vi "Save Measurement.vi"(1 "Measurement Config":T1, 2 "Experiment Config":T2, 4 "DMM Value":dbl, 5 "DMM 2 Value":dbl, 6 "Diode PS Voltage":dbl, 7 "Diode PS Current":dbl, 8 "error in":errorcluster, 9 "Trace Number":u64, 10 "Measurement Timestamp":timestamp, 11 "Trace":waveform(dbl)) -> (0 "error out":errorcluster)   [LabVIEW 2020]
uses:
  Typedefs/Experiment Config Control.ctl
  Typedefs/Measurement Config.ctl
  <vilib>/Utility/file.llb/Write Delimited Spreadsheet (string).vi
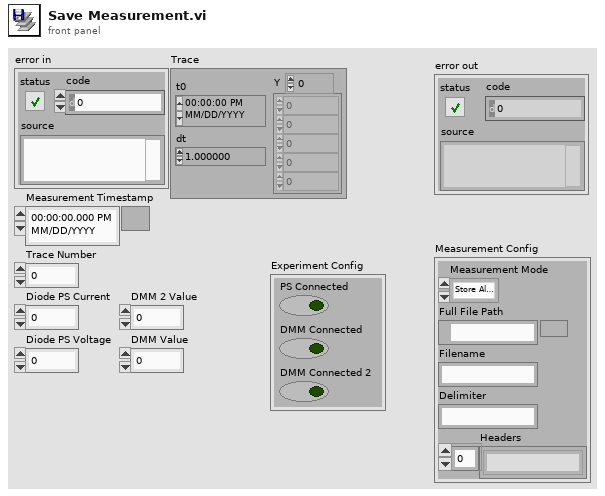
[diagram p1: front panel]
types:
  T1 = typedef "Measurement Config.ctl" = cluster{"Measurement Mode":enum16{"Store All Traces in Single File", "Store Average/Std. Dev. for each Point", "Store All Traces in Separate Files"}, "Full File Path":path, "Filename":string, "Delimiter":string, "Headers":string[]}
  T2 = typedef "Experiment Config Control.ctl" = cluster{"PS Connected":bool, "DMM Connected":bool, "DMM Connected 2":bool}
  T3 = enum16{"Store All Traces in Single File", "Store Average/Std. Dev. for each Point", "Store All Traces in Separate Files"}
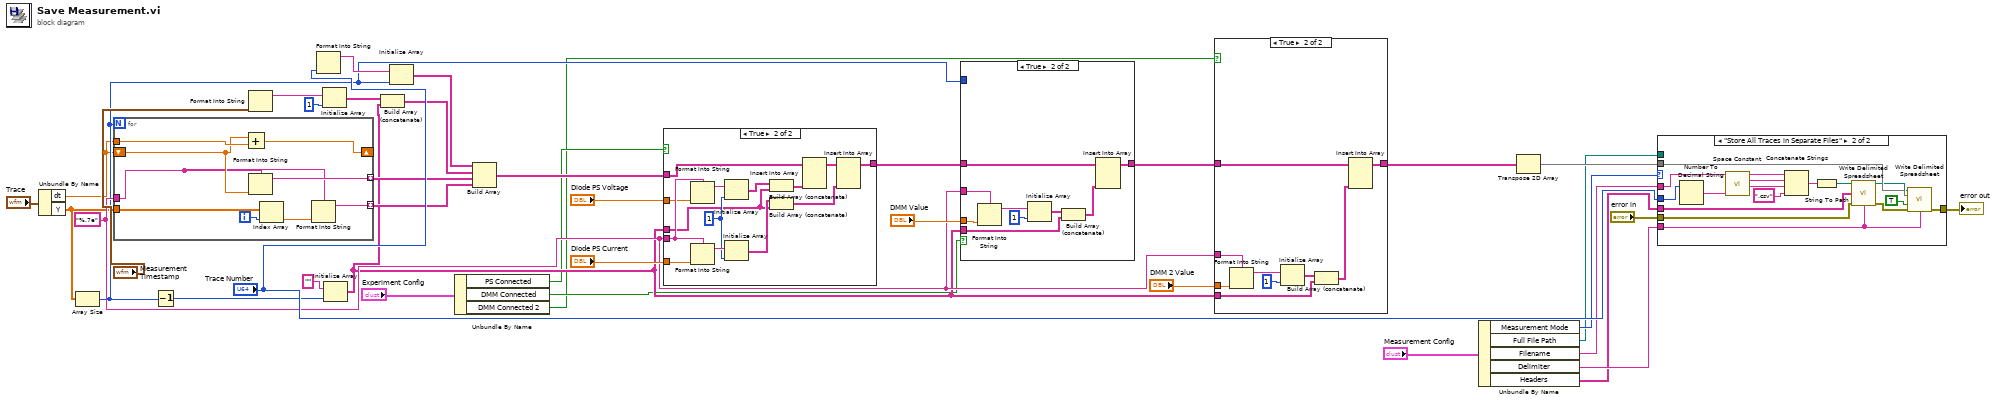
[diagram p0: block diagram]
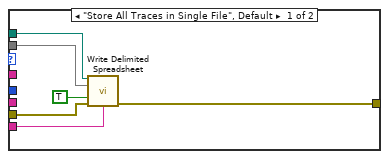
[diagram p3: hidden frame]
diagram:
  w17 = "%.7e"
  n1 = Unbundle By Name("Trace") -> ("dt"=w12:dbl, "Y"=w11:dbl[])
  n2 = Array Size(array=w11) -> (size(s)=w13:i32)
  n3 = for {
    N: w13 -> [_]
    shift-right: [w47] -> _
    shift-left: w12 -> [w46]
    tunnel: w12 -> [w48]
    tunnel: w11 -> [w42]
    tunnel: [w44] -> w26 mode=indexing
    tunnel: [w43] -> w27 mode=indexing
    tunnel: w17 -> [w40]
    i -> [w45]
    n4 = Add(x=w46, y=w48) -> (x+y=w47:dbl)
    n5 = Format Into String(format string=w40, w46) -> (resulting string=w43:string)  [unwired: 2 in, 1 out]
    n6 = Index Array(array=w42, index=w45) -> (element=w41:dbl)
    n7 = Format Into String(format string=w40, w41) -> (resulting string=w44:string)  [unwired: 2 in, 1 out]
  }
  n8 = Decrement(x=w13) -> (x-1=w21:i32)
  n9 = Format Into String("Measurement Timestamp") -> (resulting string=w29:string)  [unwired: 3 in, 1 out]
  n10 = Format Into String("Trace Number") -> (resulting string=w30:string)  [unwired: 3 in, 1 out]
  n11 = Initialize Array(w29, 1) -> (w19:string[])
  n12 = Initialize Array("", w21) -> (w16:string[])
  n13 = Build Array (concatenate)(w19, w16) -> (w18:string[])
  n14 = Initialize Array(w30, w13) -> (w28:string[])
  n15 = Unbundle By Name("Experiment Config") -> ("PS Connected"=w9:bool, "DMM Connected"=w8:bool, "DMM Connected 2"=w7:bool)
  n16 = Build Array(w28, w18, w27, w26) -> (w24:string[][])
  n17 = case shown="True" w9 {
    tunnel: w17 -> [_ w63]
    tunnel: "Diode PS Voltage" -> [_ w62]
    tunnel: "Diode PS Current" -> [_ w61]
    tunnel: w24 -> [w49 w58]
    tunnel: [w49 w56] -> w23
    tunnel: w16 -> [_ w50]
    frame False {
    }
    frame True {
      w55 = 1
      n18 = Format Into String(format string=w63, w62) -> (resulting string=w59:string)  [unwired: 2 in, 1 out]
      n19 = Format Into String(format string=w63, w61) -> (resulting string=w60:string)  [unwired: 2 in, 1 out]
      n20 = Initialize Array(w59, w55) -> (w54:string[])
      n21 = Initialize Array(w60, w55) -> (w52:string[])
      n22 = Build Array (concatenate)(w54, w50) -> (w53:string[])
      n23 = Build Array (concatenate)(w52, w50) -> (w51:string[])
      n24 = Insert Into Array(array=w58, new element=w53) -> (w57:string[][])  [unwired: 2 in]
      n25 = Insert Into Array(array=w57, new element=w51) -> (w56:string[][])  [unwired: 2 in]
    }
  }
  n26 = case shown="True" w8 {
    tunnel: w17 -> [_ w73]
    tunnel: "DMM Value" -> [_ w72]
    tunnel: w13 -> [_ _]
    tunnel: w23 -> [w64 w70]
    tunnel: [w64 w69] -> w15
    tunnel: w16 -> [_ w66]
    frame False {
    }
    frame True {
      n27 = Format Into String(format string=w73, w72) -> (resulting string=w71:string)  [unwired: 2 in, 1 out]
      n28 = Initialize Array(w71, 1 ("dimension size")) -> (w67:string[])
      n29 = Build Array (concatenate)(w67, w66) -> (w65:string[])
      n30 = Insert Into Array(array=w70, new element=w65) -> (w69:string[][])  [unwired: 2 in]
    }
  }
  n31 = case shown="True" w7 {
    tunnel: w17 -> [_ w83]
    tunnel: w16 -> [_ w80]
    tunnel: w15 -> [w74 w77]
    tunnel: [w74 w76] -> w14
    tunnel: "DMM 2 Value" -> [_ w75]
    frame False {
    }
    frame True {
      n32 = Format Into String(format string=w83, w75) -> (resulting string=w82:string)  [unwired: 2 in, 1 out]
      n33 = Initialize Array(w82, 1 ("dimension size")) -> (w79:string[])
      n34 = Build Array (concatenate)(w79, w80) -> (w78:string[])
      n35 = Insert Into Array(array=w77, new element=w78) -> (w76:string[][])  [unwired: 2 in]
    }
  }
  n36 = Unbundle By Name("Measurement Config") -> ("Measurement Mode"=w6:T3, "Full File Path"=w5:path, "Filename"=w4:string, "Delimiter"=w3:string, "Headers"=w1:string[])
  n37 = Transpose 2D Array(2D array=w14) -> (transposed array=w25:string[][])
  n38 = case shown="\"Store All Traces in Separate Files\"" w6 {
    tunnel: w25 -> [w88 w97]
    tunnel: w5 -> [w87 _]
    tunnel: w3 -> [w86 w92]
    tunnel: [w85 w93] -> w35
    tunnel: "error in" -> [w84 w98]
    tunnel: "Trace Number" -> [_ w104]
    tunnel: w4 -> [_ w91]
    tunnel: w1 -> [_ w90]
    frame "Store All Traces in Single File", Default {
      n39 = call-poly <vilib>:"Write Delimited Spreadsheet.vi"("file path (dialog if empty)"=w87, "2D data"=w88, "append to file? (new file:F)"=TRUE, "error in (no error)"=w84, "delimiter (\\t)"=w86) -> ("error out"=w85:errorcluster)  [unwired: 9 in, 1 out]
    }
    frame "Store All Traces in Separate Files" {
      n40 = Number To Decimal String(number=w104) -> (decimal integer string=w102:string)  [unwired: 1 in]
      n41 = call <vilib>:"Space Constant.vi"() -> ("String"=w103:string)
      n42 = Concatenate Strings(w91, w103, w102, ".csv" ("string")) -> (w100:string)
      n43 = String To Path(string=w100) -> (path=w99:path)
      n44 = call-poly <vilib>:"Write Delimited Spreadsheet.vi"("file path (dialog if empty)"=w99, "1D data"=w90, "error in (no error)"=w98, "delimiter (\\t)"=w92) -> ("new file path (Not A Path if cancelled)"=w96:path, "error out"=w94:errorcluster)  [unwired: 10 in]
      n45 = call-poly <vilib>:"Write Delimited Spreadsheet.vi"("file path (dialog if empty)"=w96, "2D data"=w97, "append to file? (new file:F)"=TRUE, "error in (no error)"=w94, "delimiter (\\t)"=w92) -> ("error out"=w93:errorcluster)  [unwired: 9 in, 1 out]
    }
  }
  "error out" <- w35
